vi "Write CRD Heater.vi"(8 "error in (no error)":errorcluster, 10 "Controller.lvlib:Heater Data":refnum<class "Heater Data.lvclass">, 11 "SOAP Data in":refnum<class "SOAP Data.lvclass">) -> (0 "error out":errorcluster, 3 "SOAP Data out":refnum<class "SOAP Data.lvclass">)   [LabVIEW 2017, in "Controller.lvlib" / "SOAP Data.lvclass"]
uses:
  SOAP Data.lvclass
  Heater Data/Heater Data.lvclass
  SOAP Data.lvclass/SOAP Data.ctl
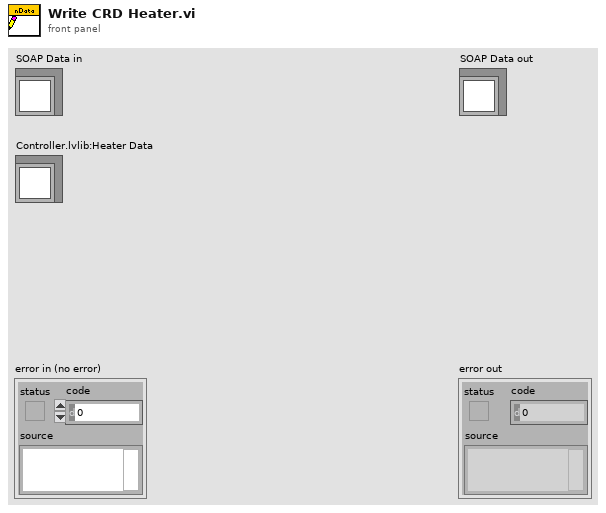
[diagram p1: front panel]
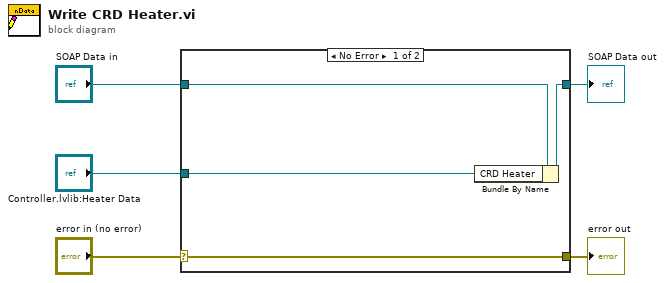
[diagram p0: block diagram]
diagram:
  n1 = case shown="No Error" "error in (no error)" {
    selector: "error in (no error)" -> [w9 w10]
    tunnel: [w9 w10] -> w4
    tunnel: [w7 w11] -> w2
    tunnel: "SOAP Data in" -> [w8 w11]
    tunnel: "Controller.lvlib:Heater Data" -> [w6 _]
    frame No Error {
      n2 = Bundle By Name(cluster=w8, "CRD Heater"=w6) -> (w7:refnum<class "SOAP Data.lvclass">)
    }
    frame Error {
    }
  }
  "error out" <- w4
  "SOAP Data out" <- w2
